vi "Control_Layer.vi"(8 "stop":bool, 10 "Active Axes":bool[](array[boolean]), 11 "Angles":dbl[](array[numeric])=[0.0, 0.0, 0.0, 0.0, 0.0]) -> ()   [LabVIEW 2014]
uses:
  <vilib>/Platform/TimedLoop/XDataNode/timing_clust.ctl
  <vilib>/Platform/TimedLoop/XDataNode/nitl_modes.ctl
  <vilib>/Platform/TimedLoop/XDataNode/wakeup.ctl
  <vilib>/FPGAPlugInAG/cRIO-9068/niLvFpga_Open_cRIO-9068.vi
  <vilib>/rvi/interface/common/dynamic/niFpgaDynamicAddResources.vi
  <vilib>/Utility/error.llb/Error Cluster From Error Code.vi
  <vilib>/rvi/errors/niLvFpgaAdjustHostInterfaceError.vi
  <vilib>/addons/control/pid/pid.llb/PID (DBL).vi
  <vilib>/FPGAPlugInAG/Dynamic/niLvFpga_Close_Dynamic.vi
  <vilib>/rvi/interface/nirviOpenFPGA/nirviOpenFPGA.xnode
  FPGA Bitfiles/MotorControl_FPGATarget_RobotControl_55TRSUIRMao.lvbitx
  <vilib>/rvi/interface/nirviReadWriteControl/nirviReadWriteControl.xnode
  <vilib>/Platform/TimedLoop/XDataNode/XDataNode.xnode
  <vilib>/rvi/interface/nirviCloseFPGA/nirviCloseFPGA.xnode
  <vilib>/rvi/interface/Simulation/niFpgaSimulationCallBeginRW.vi
  NiFpgaLv.dll
  <vilib>/addons/control/pid/NI_PID_pid.lvlib
  <vilib>/Platform/TimedLoop/XDataNode/XDNodeRunTimeDep.lvlib
panel:
  in  "Trapezoidal Move":bool
  out "appended array":dbl[][](array[numeric])
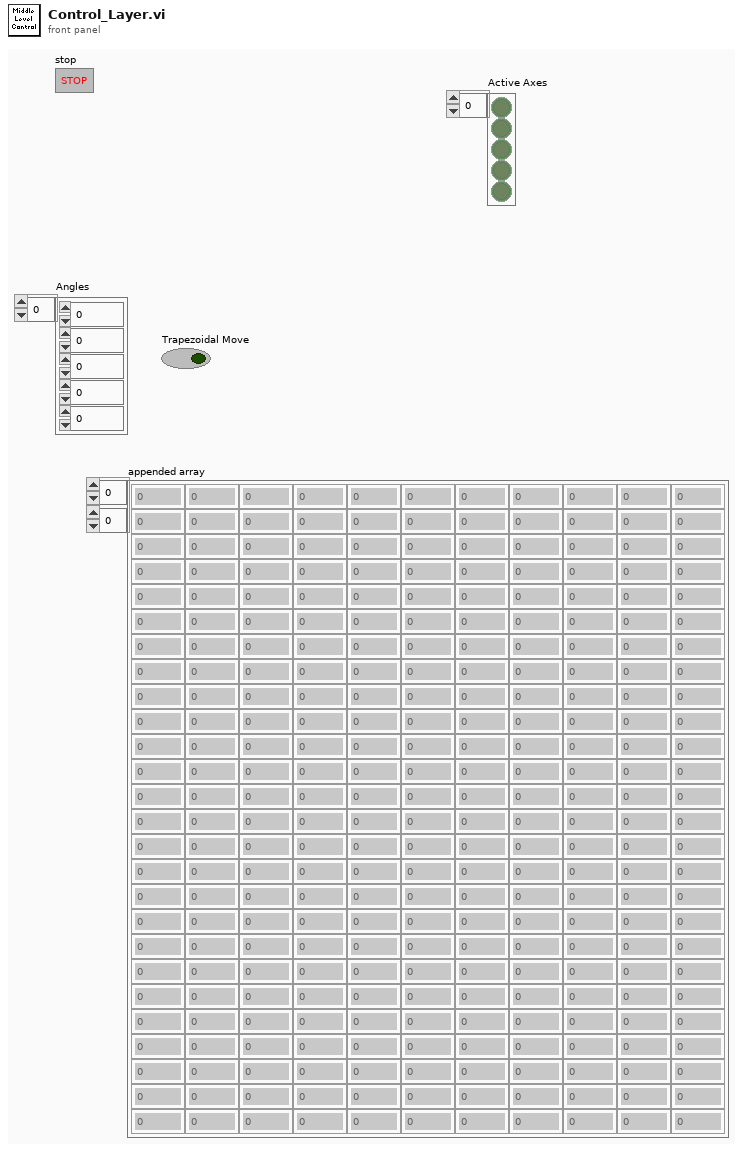
[diagram p1: front panel]
types:
  T1 = typedef "XDNodeRunTimeDep.lvlib/timing_clust.ctl" = cluster{"Expected End [f-1]":u64, "Actual End [f-1]":u64, "Finished Late? [f-1]":bool, "Expected End [i-1]":u64, "Actual End [i-1]":u64, "Finished Late? [i-1]":bool, "Expected Start [i]":u64, "Actual Start [i]":u64, "Expected Start [f]":u64, "Actual Start [f]":u64, "Source Name":string, "Structure Name":string, "Period":i64, "Deadline":i64, "Offset":i64, "Start":i64, "Priority":i32, "Timeout":i32, "Mode":T2, "Wakeup Reason":T3, "Error":errorcluster, "Source Type":string, "Secondary Source Type":string, "Global End Time":u64, "Global Start Time":u64, "Frame Duration":u64, "Iteration Duration":u64, "Assigned CPU":i32, "I/O Scan Engine Mode":u32}
  T2 = typedef "XDNodeRunTimeDep.lvlib/nitl_modes.ctl" = enum32{"No Change", "Process missed periods, maintain original phase", "Discard missed periods, maintain original phase", "Process missed periods, ignore original phase", "Discard missed periods, ignore original phase"}
  T3 = typedef "XDNodeRunTimeDep.lvlib/wakeup.ctl" = enum32{"Normal", "Aborted", "Asynchronous wakeup", "Timing source error", "Timed loop error", "Timeout"}
  T4 = cluster{"Motor 1 Variables":cluster{"Motor 1 P Gains":cluster{"proportional gain (Kc)":dbl, "integral time (Ti, min)":dbl, "derivative time (Td, min)":dbl}, "Motor 1 V Gains":cluster{"proportional gain (Kc)":dbl, "integral time (Ti, min)":dbl, "derivative time (Td, min)":dbl}, "Velocity Limits":cluster{"output high":dbl, "output low":dbl}, "Duty Cycle Limits":cluster{"output high":dbl, "output low":dbl}}, "Motor 2 Variables":cluster{"Motor 2 P Gains":cluster{"proportional gain (Kc)":dbl, "integral time (Ti, min)":dbl, "derivative time (Td, min)":dbl}, "Motor 2 V Gains":cluster{"proportional gain (Kc)":dbl, "integral time (Ti, min)":dbl, "derivative time (Td, min)":dbl}, "Velocity Limits":cluster{"output high":dbl, "output low":dbl}, "Duty Cycle Limits":cluster{"output high":dbl, "output low":dbl}}, "Motor 3 Variables":cluster{"Motor 3 P Gains":cluster{"proportional gain (Kc)":dbl, "integral time (Ti, min)":dbl, "derivative time (Td, min)":dbl}, "Motor 3 V Gains":cluster{"proportional gain (Kc)":dbl, "integral time (Ti, min)":dbl, "derivative time (Td, min)":dbl}, "Velocity Limits":cluster{"output high":dbl, "output low":dbl}, "Duty Cycle Limits":cluster{"output high":dbl, "output low":dbl}}, "Motor 4 Variables":cluster{"Motor 4 P Gains":cluster{"proportional gain (Kc)":dbl, "integral time (Ti, min)":dbl, "derivative time (Td, min)":dbl}, "Motor 4 V Gains":cluster{"proportional gain (Kc)":dbl, "integral time (Ti, min)":dbl, "derivative time (Td, min)":dbl}, "Velocity Limits":cluster{"output high":dbl, "output low":dbl}, "Duty Cycle Limits":cluster{"output high":dbl, "output low":dbl}}, "Motor 5 Variables":cluster{"Motor 5 P Gains":cluster{"proportional gain (Kc)":dbl, "integral time (Ti, min)":dbl, "derivative time (Td, min)":dbl}, "Motor 5 V Gains":cluster{"proportional gain (Kc)":dbl, "integral time (Ti, min)":dbl, "derivative time (Td, min)":dbl}, "Velocity Limits":cluster{"output high":dbl, "output low":dbl}, "Duty Cycle Limits":cluster{"output high":dbl, "output low":dbl}}}
  T5 = cluster{"Motor 1 P Gains":cluster{"proportional gain (Kc)":dbl, "integral time (Ti, min)":dbl, "derivative time (Td, min)":dbl}, "Motor 1 V Gains":cluster{"proportional gain (Kc)":dbl, "integral time (Ti, min)":dbl, "derivative time (Td, min)":dbl}, "Velocity Limits":cluster{"output high":dbl, "output low":dbl}, "Duty Cycle Limits":cluster{"output high":dbl, "output low":dbl}}
  T6 = cluster{"proportional gain (Kc)":dbl, "integral time (Ti, min)":dbl, "derivative time (Td, min)":dbl}
  T7 = cluster{"Motor 2 P Gains":cluster{"proportional gain (Kc)":dbl, "integral time (Ti, min)":dbl, "derivative time (Td, min)":dbl}, "Motor 2 V Gains":cluster{"proportional gain (Kc)":dbl, "integral time (Ti, min)":dbl, "derivative time (Td, min)":dbl}, "Velocity Limits":cluster{"output high":dbl, "output low":dbl}, "Duty Cycle Limits":cluster{"output high":dbl, "output low":dbl}}
  T8 = cluster{"Motor 3 P Gains":cluster{"proportional gain (Kc)":dbl, "integral time (Ti, min)":dbl, "derivative time (Td, min)":dbl}, "Motor 3 V Gains":cluster{"proportional gain (Kc)":dbl, "integral time (Ti, min)":dbl, "derivative time (Td, min)":dbl}, "Velocity Limits":cluster{"output high":dbl, "output low":dbl}, "Duty Cycle Limits":cluster{"output high":dbl, "output low":dbl}}
  T9 = cluster{"Motor 4 P Gains":cluster{"proportional gain (Kc)":dbl, "integral time (Ti, min)":dbl, "derivative time (Td, min)":dbl}, "Motor 4 V Gains":cluster{"proportional gain (Kc)":dbl, "integral time (Ti, min)":dbl, "derivative time (Td, min)":dbl}, "Velocity Limits":cluster{"output high":dbl, "output low":dbl}, "Duty Cycle Limits":cluster{"output high":dbl, "output low":dbl}}
  T10 = cluster{"Motor 5 P Gains":cluster{"proportional gain (Kc)":dbl, "integral time (Ti, min)":dbl, "derivative time (Td, min)":dbl}, "Motor 5 V Gains":cluster{"proportional gain (Kc)":dbl, "integral time (Ti, min)":dbl, "derivative time (Td, min)":dbl}, "Velocity Limits":cluster{"output high":dbl, "output low":dbl}, "Duty Cycle Limits":cluster{"output high":dbl, "output low":dbl}}
  T11 = cluster{"Position (Degrees)":dbl, "Numeric":dbl, "Acceleration":dbl, "Cruise_Velocity":dbl, "Deceleration":dbl, "Time_Accelerate":dbl, "Time_2":dbl, "Time_Total":dbl}
  T12 = cluster{"Acceleration":dbl, "Cruise_Velocity":dbl, "Deceleration":dbl, "Time_Accelerate":dbl, "Time_2":dbl, "Time_Total":dbl}
  T13 = cluster{dbl, "Numeric":dbl, "Acceleration":dbl, "Cruise_Velocity":dbl, "Deceleration":dbl, "Time_Accelerate":dbl, "Time_2":dbl, "Time_Total":dbl}
  T14 = cluster{dbl, dbl, "Acceleration":dbl, "Cruise_Velocity":dbl, "Deceleration":dbl, "Time_Accelerate":dbl, "Time_2":dbl, "Time_Total":dbl}
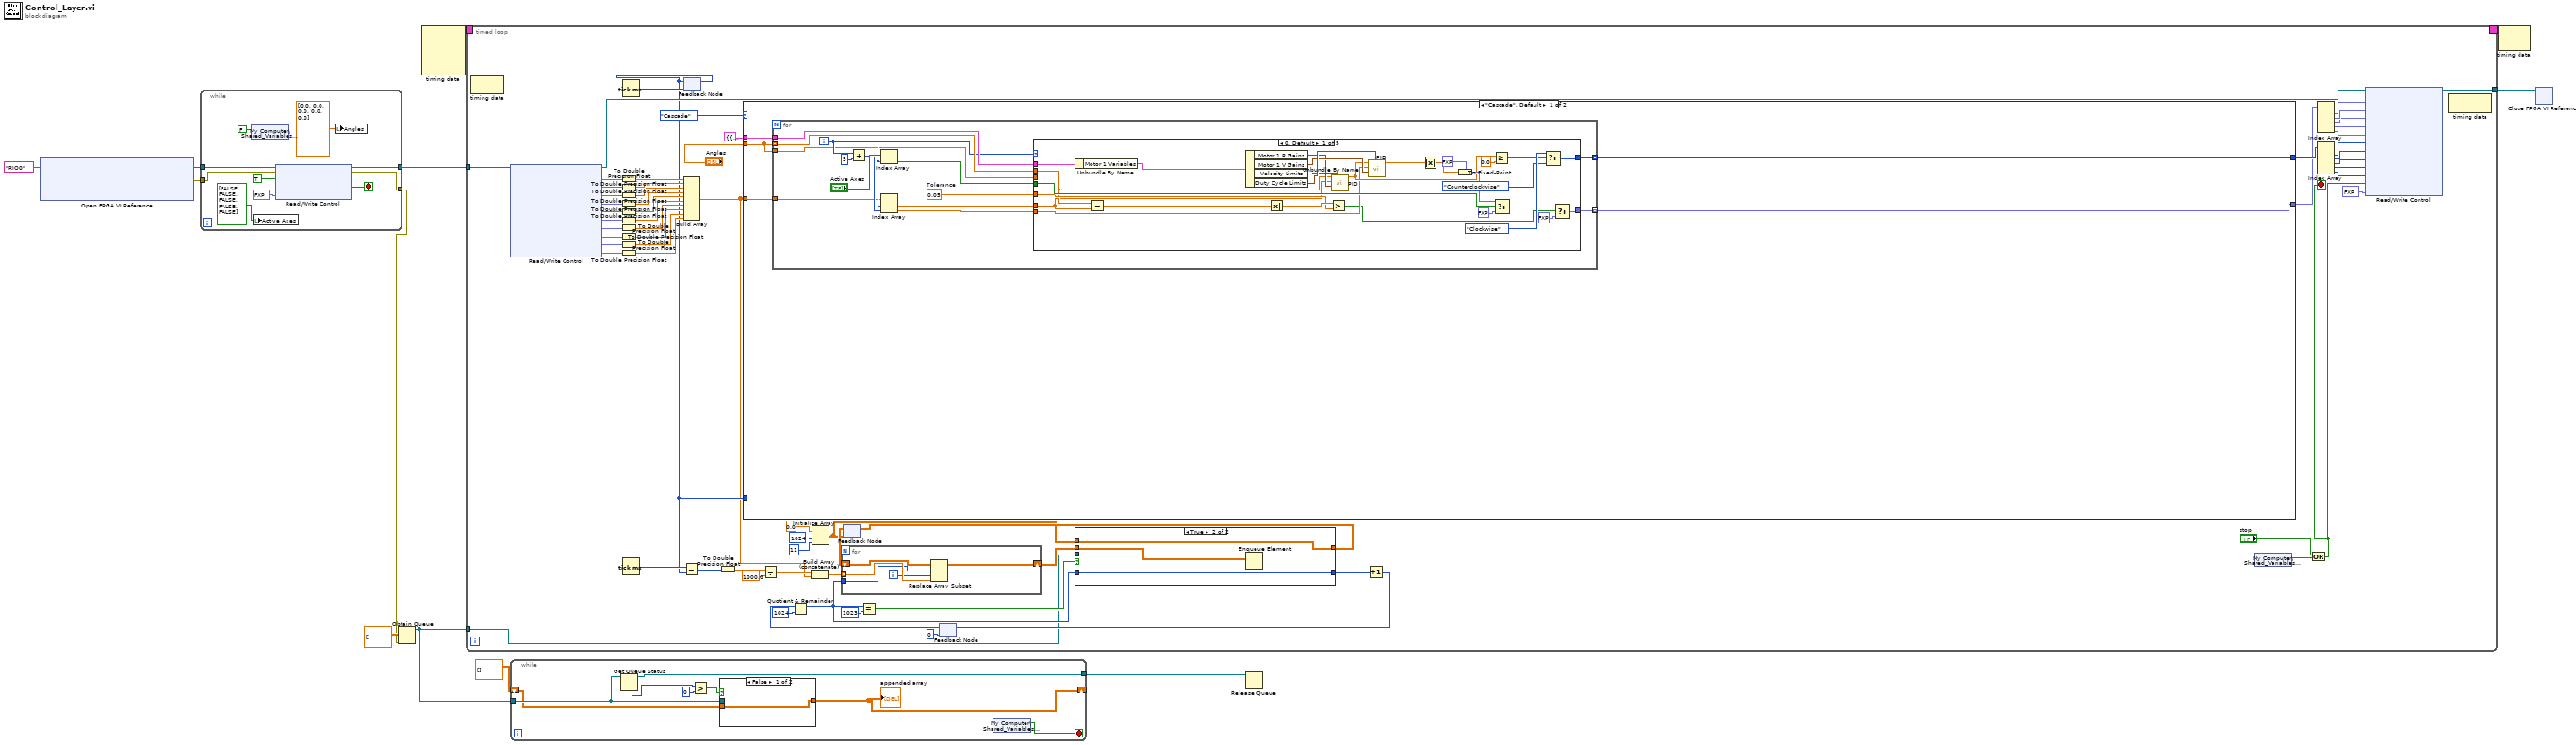
[diagram p0: block diagram]
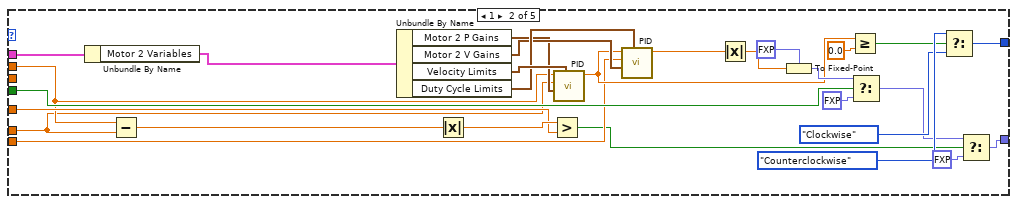
[diagram p2: hidden frame]
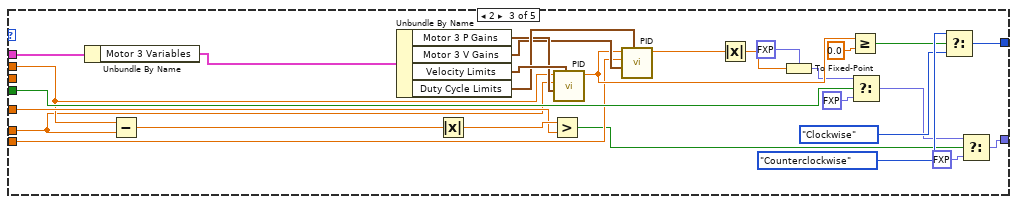
[diagram p3: hidden frame]
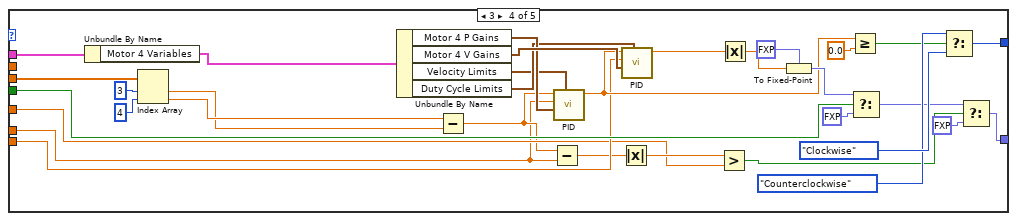
[diagram p4: hidden frame]
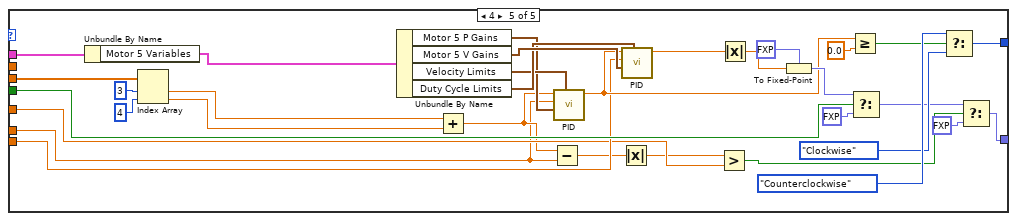
[diagram p5: hidden frame]
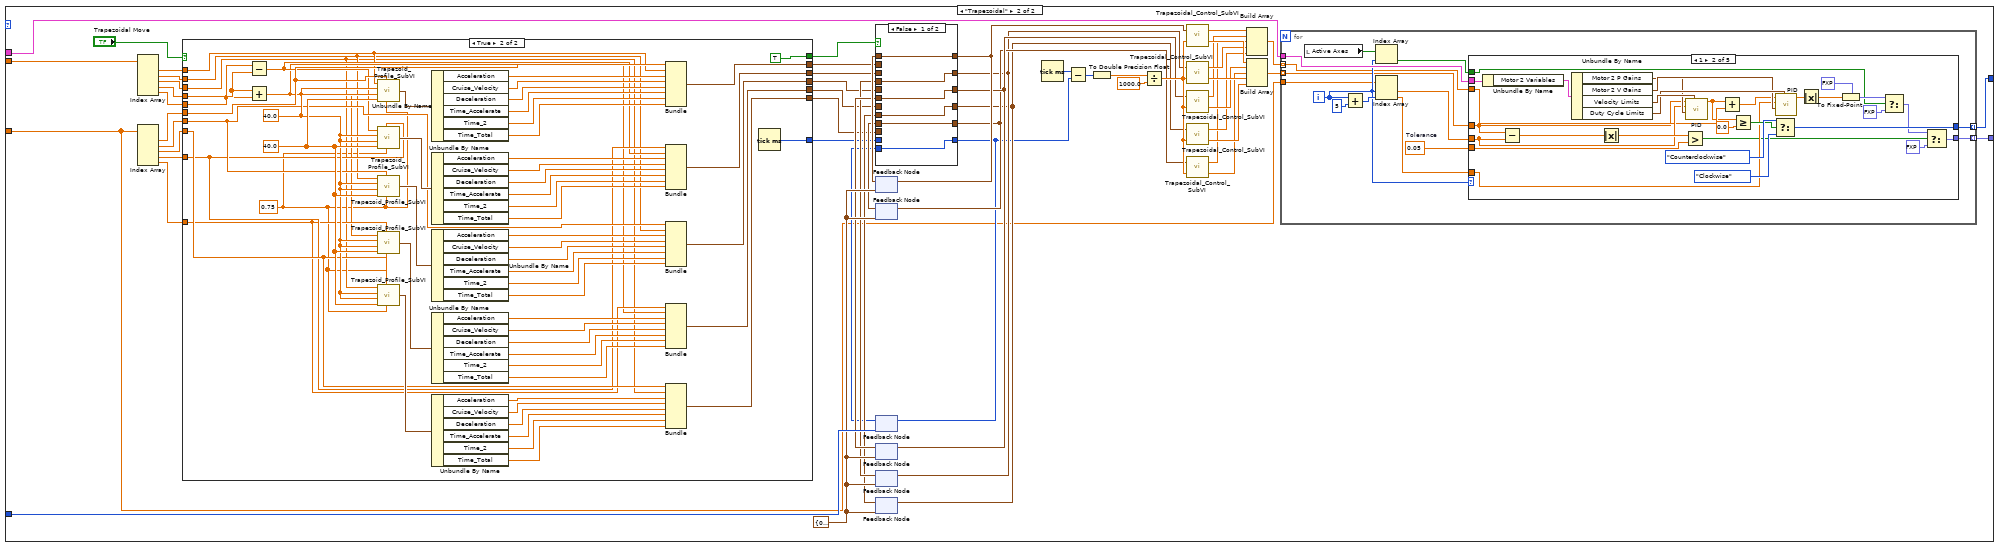
[diagram p6: hidden frame]
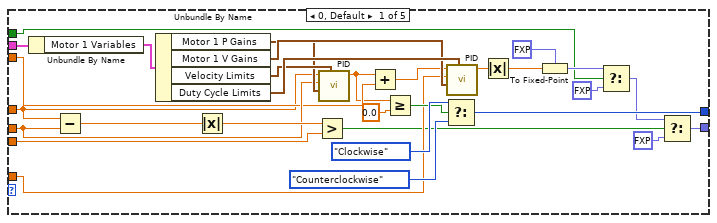
[diagram p7: hidden frame]
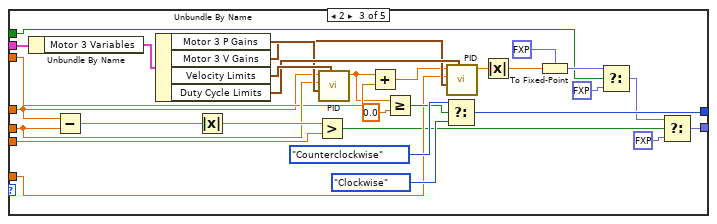
[diagram p8: hidden frame]
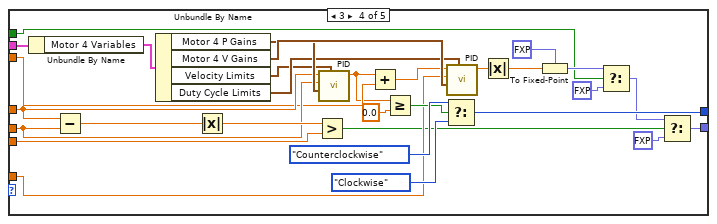
[diagram p9: hidden frame]
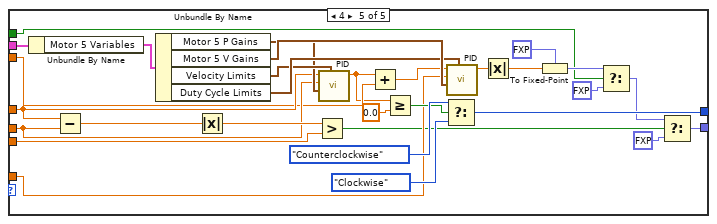
[diagram p10: hidden frame]
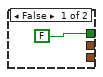
[diagram p11: hidden frame]
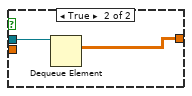
[diagram p14: hidden frame]
diagram:
  n1 = xnode "Open FPGA VI Reference"("resource name"=tag "RIO0") -> ("FPGA VI Reference Out"=w11:refnum<k20>, "error out"=w2:errorcluster)  [unwired: 1 in]
  n2 = while {
    tunnel: w11 -> [w22]
    tunnel: [w19] -> w6
    tunnel: w2 -> [w14]
    tunnel: [w13] -> w1
    stop <- w20 stop-if-true
    n3 = shared-variable "My Computer\\Shared_Variables.lvlib\\Stop"(FALSE ("Stop")) -> ()  [unwired: 1 in, 1 out]
    n4 = local write "Active Axes"(bool[] [FALSE, FALSE, FALSE, FALSE, FALSE] ("Active Axes")) -> ()
    n5 = xnode "Read/Write Control"("FPGA VI Reference In"=w22, "error in"=w14, "Go"=TRUE, "Velocity Interval (uSec)"=fxp<+/-,40,24> 5000.0) -> ("FPGA VI Reference Out"=w19:refnum<k20>, "error out"=w13:errorcluster, "Homed"=w20:bool)
    n6 = local write "Angles"(dbl[] [0.0, 0.0, 0.0, 0.0, 0.0] ("Angles")) -> ()
  }
  n7 = Obtain Queue(element data type=dbl[][] [], error in (no error)=w1) -> (queue out=w9:refnum<queue>)  [unwired: 3 in, 2 out]
  n8 = node-c288() -> (w4:T1)  [unwired: 4 in]
  n9 = timed-loop {
    tunnel: [w89] -> w12
    tunnel: w6 -> [w87]
    tunnel: w9 -> [w46]
    timing: w4 -> [_]
    timing-out: [_] -> w3
    stop <- w25 stop-if-true
    n10 = node-c288() -> ()  [unwired: 1 in, 1 out]
    n11 = xnode "Read/Write Control"("FPGA VI Reference In"=w87) -> ("FPGA VI Reference Out"=w82:refnum<k20>, "Position (Degrees)"=w81:fxp<+/-,40,24>, "Position (Degrees) 2"=w80:fxp<+/-,40,24>, "Position (Degrees) 3"=w79:fxp<+/-,40,24>, "Position (Degrees) 4"=w78:fxp<+/-,40,24>, "Position (Degrees) 5"=w77:fxp<+/-,40,24>, "Velocity (Degrees/Second)"=w76:fxp<+/-,40,24>, "Velocity (Degrees/Second) 2"=w75:fxp<+/-,40,24>, "Velocity (Degrees/Second) 3"=w74:fxp<+/-,40,24>, "Velocity (Degrees/Second) 4"=w73:fxp<+/-,40,24>, "Velocity (Degrees/Second) 5"=w72:fxp<+/-,40,24>)  [unwired: 1 in, 1 out]
    n12 = To Double Precision Float(number=w81) -> (double precision float=w64:dbl)
    n13 = To Double Precision Float(number=w80) -> (double precision float=w63:dbl)
    n14 = To Double Precision Float(number=w79) -> (double precision float=w62:dbl)
    n15 = To Double Precision Float(number=w78) -> (double precision float=w61:dbl)
    n16 = To Double Precision Float(number=w77) -> (double precision float=w60:dbl)
    n17 = To Double Precision Float(number=w76) -> (double precision float=w59:dbl)
    n18 = To Double Precision Float(number=w75) -> (double precision float=w58:dbl)
    n19 = To Double Precision Float(number=w74) -> (double precision float=w57:dbl)
    n20 = To Double Precision Float(number=w73) -> (double precision float=w56:dbl)
    n21 = To Double Precision Float(number=w72) -> (double precision float=w55:dbl)
    n22 = Tick Count (ms)() -> (millisecond timer value=w44:u32)
    n23 = Tick Count (ms)() -> (millisecond timer value=w86:u32)
    n24 = Build Array(w64, w63, w62, w61, w60, w59, w58, w57, w56, w55) -> (w39:dbl[])
    n25 = feedback #1(w44) -> (w43:u32)
    n26 = Subtract(x=w86, y=w43) -> (x-y=w85:u32)
    n27 = feedback-in #1(w43) -> ()
    n28 = To Double Precision Float(number=w85) -> (double precision float=w83:dbl)
    n29 = case shown="\"Cascade\", Default" enum16{"Cascade", "Trapezoidal"}."Cascade" {
      tunnel: w43 -> [_ w314]
      tunnel: T4 {"Motor 1 Variables"={"Motor 1 P Gains"={"proportional gain (Kc)"=3.0, "integral time (Ti, min)"=0.0, "derivative time (Td, min)"=0.0}, "Motor 1 V Gains"={"proportional gain (Kc)"=0.001, "integral time (Ti, min)"=0.0001, "derivative time (Td, min)"=0.0}, "Velocity Limits"={"output high"=40.0, "output low"=-40.0}, "Duty Cycle Limits"={"output high"=0.6, "output low"=-0.6}}, "Motor 2 Variables"={"Motor 2 P Gains"={"proportional gain (Kc)"=2.0, "integral time (Ti, min)"=0.0, "derivative time (Td, min)"=0.0}, "Motor 2 V Gains"={"proportional gain (Kc)"=0.002, "integral time (Ti, min)"=0.0003, "derivative time (Td, min)"=0.0}, "Velocity Limits"={"output high"=40.0, "output low"=-40.0}, "Duty Cycle Limits"={"output high"=0.6, "output low"=-0.6}}, "Motor 3 Variables"={"Motor 3 P Gains"={"proportional gain (Kc)"=2.0, "integral time (Ti, min)"=0.0, "derivative time (Td, min)"=0.0}, "Motor 3 V Gains"={"proportional gain (Kc)"=0.004, "integral time (Ti, min)"=0.0003, "derivative time (Td, min)"=0.0}, "Velocity Limits"={"output high"=40.0, "output low"=-40.0}, "Duty Cycle Limits"={"output high"=0.6, "output low"=-0.6}}, "Motor 4 Variables"={"Motor 4 P Gains"={"proportional gain (Kc)"=3.0, "integral time (Ti, min)"=0.0, "derivative time (Td, min)"=0.0}, "Motor 4 V Gains"={"proportional gain (Kc)"=0.0004, "integral time (Ti, min)"=0.0001, "derivative time (Td, min)"=0.0}, "Velocity Limits"={"output high"=40.0, "output low"=-40.0}, "Duty Cycle Limits"={"output high"=0.6, "output low"=-0.6}}, "Motor 5 Variables"={"Motor 5 P Gains"={"proportional gain (Kc)"=3.0, "integral time (Ti, min)"=0.0, "derivative time (Td, min)"=0.0}, "Motor 5 V Gains"={"proportional gain (Kc)"=0.0004, "integral time (Ti, min)"=0.0001, "derivative time (Td, min)"=0.0}, "Velocity Limits"={"output high"=40.0, "output low"=-40.0}, "Duty Cycle Limits"={"output high"=0.6, "output low"=-0.6}}} ("Motor Variables") -> [w95 w275]
      tunnel: "Angles" -> [w94 w282]
      tunnel: w39 -> [w96 w276]
      tunnel: [w93 w269] -> w38
      tunnel: [w92 w270] -> w32
      frame "Cascade", Default {
        n30 = for {
          tunnel: w94 -> [w109] mode=indexing
          tunnel: w96 -> [w100]
          tunnel: w95 -> [w110]
          tunnel: [w108] -> w93 mode=indexing
          tunnel: [w107] -> w92 mode=indexing
          tunnel: w94 -> [w98]
          i -> [w102]
          w97 = 0.05  # Tolerance
          n31 = Add(x=w102, y=5) -> (x+y=w103:i32)
          n32 = Index Array(array="Active Axes", index=w102) -> (element=w105:bool)
          n33 = Index Array(array=w100, index #1=w102, index #2=w103) -> (element #1=w101:dbl, element #2=w99:dbl)
          n34 = case shown="0, Default" w102 {
            tunnel: w110 -> [w124 w153 w180 w213 w246]
            tunnel: w109 -> [w112 w140 w168 _ _]
            tunnel: [w123 w152 w179 w212 w245] -> w108
            tunnel: [w116 w141 w169 w197 w230] -> w107
            tunnel: w105 -> [w122 w151 w178 w211 w244]
            tunnel: w101 -> [w111 w139 w167 w195 w228]
            tunnel: w99 -> [w120 w148 w176 w209 w242]
            tunnel: w98 -> [_ _ _ w208 w239]
            tunnel: w97 -> [w114 w143 w171 w199 w234]
            frame 0, Default {
              n35 = Unbundle By Name(w124) -> ("Motor 1 Variables"=w125:T5)
              n36 = Subtract(x=w112, y=w111) -> (x-y=w113:dbl)
              n37 = Unbundle By Name(w125) -> ("Motor 1 P Gains"=w130:T6, "Motor 1 V Gains"=w131:T6, "Velocity Limits"=w132:cluster{"output high":dbl, "output low":dbl}, "Duty Cycle Limits"=w133:cluster{"output high":dbl, "output low":dbl})
              n38 = Absolute Value(x=w113) -> (abs(x)=w115:dbl)
              n39 = Greater?(x=w115, y=w114) -> (0:w118:bool)
              n40 = call-poly <vilib>:"PID.vi"("output range"=w132, "PID gains"=w130, "process variable"=w111, "setpoint"=w112) -> ("output"=w127:dbl)  [unwired: 6 in, 1 out]
              n41 = call-poly <vilib>:"PID.vi"("output range"=w133, "PID gains"=w131, "process variable"=w120, "setpoint"=w127) -> ("output"=w128:dbl)  [unwired: 6 in, 1 out]
              n42 = Absolute Value(x=w128) -> (abs(x)=w129:dbl)
              n43 = To Fixed-Point(fixed-point type=fxp<+,32,0> 0.0 ("Duty Cycle 1"), number=w129) -> (fixed-point=w135:fxp<+,32,0>)
              n44 = Greater Or Equal?(x=w127, y=0.0) -> (x >= y?=w136:bool)
              n45 = Select(t=w135, s=w122, f=fxp<+,32,0> 0.0 ("Duty Cycle 1")) -> (s? t:f=w117:fxp<+,32,0>)
              n46 = Select(t=enum8{"Clockwise", "Counterclockwise"}."Clockwise" ("Mod1/Drive Direction"), s=w136, f=enum8{"Clockwise", "Counterclockwise"}."Counterclockwise" ("Mod1/Drive Direction")) -> (s? t:f=w123:enum8{"Clockwise", "Counterclockwise"})
              n47 = Select(t=w117, s=w118, f=fxp<+,32,0> 0.0 ("Duty Cycle 1")) -> (s? t:f=w116:fxp<+,32,0>)
            }
            frame 1 {
              n48 = Unbundle By Name(w153) -> ("Motor 2 Variables"=w154:T7)
              n49 = Subtract(x=w140, y=w139) -> (x-y=w145:dbl)
              n50 = Unbundle By Name(w154) -> ("Motor 2 P Gains"=w158:T6, "Motor 2 V Gains"=w159:T6, "Velocity Limits"=w161:cluster{"output high":dbl, "output low":dbl}, "Duty Cycle Limits"=w160:cluster{"output high":dbl, "output low":dbl})
              n51 = Absolute Value(x=w145) -> (abs(x)=w144:dbl)
              n52 = Greater?(x=w144, y=w143) -> (0:w146:bool)
              n53 = call-poly <vilib>:"PID.vi"("output range"=w161, "PID gains"=w158, "process variable"=w139, "setpoint"=w140) -> ("output"=w149:dbl)  [unwired: 6 in, 1 out]
              n54 = call-poly <vilib>:"PID.vi"("output range"=w160, "PID gains"=w159, "process variable"=w148, "setpoint"=w149) -> ("output"=w156:dbl)  [unwired: 6 in, 1 out]
              n55 = Absolute Value(x=w156) -> (abs(x)=w157:dbl)
              n56 = To Fixed-Point(fixed-point type=fxp<+,32,0> 0.0 ("Duty Cycle 1"), number=w157) -> (fixed-point=w163:fxp<+,32,0>)
              n57 = Greater Or Equal?(x=w149, y=0.0) -> (x >= y?=w164:bool)
              n58 = Select(t=w163, s=w151, f=fxp<+,32,0> 0.0 ("Duty Cycle 1")) -> (s? t:f=w142:fxp<+,32,0>)
              n59 = Select(t=enum8{"Clockwise", "Counterclockwise"}."Counterclockwise" ("Mod1/Drive Direction"), s=w164, f=enum8{"Clockwise", "Counterclockwise"}."Clockwise" ("Mod1/Drive Direction")) -> (s? t:f=w152:enum8{"Clockwise", "Counterclockwise"})
              n60 = Select(t=w142, s=w146, f=fxp<+,32,0> 0.0 ("Duty Cycle 1")) -> (s? t:f=w141:fxp<+,32,0>)
            }
            frame 2 {
              n61 = Unbundle By Name(w180) -> ("Motor 3 Variables"=w181:T8)
              n62 = Subtract(x=w168, y=w167) -> (x-y=w173:dbl)
              n63 = Unbundle By Name(w181) -> ("Motor 3 P Gains"=w189:T6, "Motor 3 V Gains"=w188:T6, "Velocity Limits"=w191:cluster{"output high":dbl, "output low":dbl}, "Duty Cycle Limits"=w190:cluster{"output high":dbl, "output low":dbl})
              n64 = Absolute Value(x=w173) -> (abs(x)=w172:dbl)
              n65 = Greater?(x=w172, y=w171) -> (0:w174:bool)
              n66 = call-poly <vilib>:"PID.vi"("output range"=w191, "PID gains"=w189, "process variable"=w167, "setpoint"=w168) -> ("output"=w185:dbl)  [unwired: 6 in, 1 out]
              n67 = call-poly <vilib>:"PID.vi"("output range"=w190, "PID gains"=w188, "process variable"=w176, "setpoint"=w185) -> ("output"=w186:dbl)  [unwired: 6 in, 1 out]
              n68 = Absolute Value(x=w186) -> (abs(x)=w187:dbl)
              n69 = To Fixed-Point(fixed-point type=fxp<+,32,0> 0.0 ("Duty Cycle 1"), number=w187) -> (fixed-point=w182:fxp<+,32,0>)
              n70 = Greater Or Equal?(x=w185, y=0.0) -> (x >= y?=w192:bool)
              n71 = Select(t=w182, s=w178, f=fxp<+,32,0> 0.0 ("Duty Cycle 1")) -> (s? t:f=w170:fxp<+,32,0>)
              n72 = Select(t=enum8{"Clockwise", "Counterclockwise"}."Counterclockwise" ("Mod1/Drive Direction"), s=w192, f=enum8{"Clockwise", "Counterclockwise"}."Clockwise" ("Mod1/Drive Direction")) -> (s? t:f=w179:enum8{"Clockwise", "Counterclockwise"})
              n73 = Select(t=w170, s=w174, f=fxp<+,32,0> 0.0 ("Duty Cycle 1")) -> (s? t:f=w169:fxp<+,32,0>)
            }
            frame 3 {
              n74 = Unbundle By Name(w213) -> ("Motor 4 Variables"=w214:T9)
              n75 = Index Array(array=w208, index #1=3 ("index"), index #2=4 ("index")) -> (element #1=w204:dbl, element #2=w205:dbl)
              n76 = Unbundle By Name(w214) -> ("Motor 4 P Gains"=w221:T6, "Motor 4 V Gains"=w222:T6, "Velocity Limits"=w219:cluster{"output high":dbl, "output low":dbl}, "Duty Cycle Limits"=w220:cluster{"output high":dbl, "output low":dbl})
              n77 = Subtract(x=w205, y=w204) -> (x-y=w196:dbl)
              n78 = Subtract(x=w196, y=w195) -> (x-y=w201:dbl)
              n79 = call-poly <vilib>:"PID.vi"("output range"=w219, "PID gains"=w221, "process variable"=w195, "setpoint"=w196) -> ("output"=w216:dbl)  [unwired: 6 in, 1 out]
              n80 = Absolute Value(x=w201) -> (abs(x)=w200:dbl)
              n81 = call-poly <vilib>:"PID.vi"("output range"=w220, "PID gains"=w222, "process variable"=w209, "setpoint"=w216) -> ("output"=w217:dbl)  [unwired: 6 in, 1 out]
              n82 = Greater?(x=w200, y=w199) -> (0:w202:bool)
              n83 = Absolute Value(x=w217) -> (abs(x)=w218:dbl)
              n84 = To Fixed-Point(fixed-point type=fxp<+,32,0> 0.0 ("Duty Cycle 1"), number=w218) -> (fixed-point=w224:fxp<+,32,0>)
              n85 = Greater Or Equal?(x=w216, y=0.0) -> (x >= y?=w225:bool)
              n86 = Select(t=w224, s=w211, f=fxp<+,32,0> 0.0 ("Duty Cycle 1")) -> (s? t:f=w198:fxp<+,32,0>)
              n87 = Select(t=enum8{"Clockwise", "Counterclockwise"}."Counterclockwise" ("Mod1/Drive Direction"), s=w225, f=enum8{"Clockwise", "Counterclockwise"}."Clockwise" ("Mod1/Drive Direction")) -> (s? t:f=w212:enum8{"Clockwise", "Counterclockwise"})
              n88 = Select(t=w198, s=w202, f=fxp<+,32,0> 0.0 ("Duty Cycle 1")) -> (s? t:f=w197:fxp<+,32,0>)
            }
            frame 4 {
              n89 = Unbundle By Name(w246) -> ("Motor 5 Variables"=w247:T10)
              n90 = Index Array(array=w239, index #1=3 ("index"), index #2=4 ("index")) -> (element #1=w238:dbl, element #2=w237:dbl)
              n91 = Unbundle By Name(w247) -> ("Motor 5 P Gains"=w252:T6, "Motor 5 V Gains"=w255:T6, "Velocity Limits"=w253:cluster{"output high":dbl, "output low":dbl}, "Duty Cycle Limits"=w254:cluster{"output high":dbl, "output low":dbl})
              n92 = Add(x=w238, y=w237) -> (x+y=w229:dbl)
              n93 = Subtract(x=w229, y=w228) -> (x-y=w232:dbl)
              n94 = call-poly <vilib>:"PID.vi"("output range"=w253, "PID gains"=w252, "process variable"=w228, "setpoint"=w229) -> ("output"=w249:dbl)  [unwired: 6 in, 1 out]
              n95 = Absolute Value(x=w232) -> (abs(x)=w233:dbl)
              n96 = call-poly <vilib>:"PID.vi"("output range"=w254, "PID gains"=w255, "process variable"=w242, "setpoint"=w249) -> ("output"=w250:dbl)  [unwired: 6 in, 1 out]
              n97 = Greater?(x=w233, y=w234) -> (0:w235:bool)
              n98 = Absolute Value(x=w250) -> (abs(x)=w251:dbl)
              n99 = To Fixed-Point(fixed-point type=fxp<+,32,0> 0.0 ("Duty Cycle 1"), number=w251) -> (fixed-point=w257:fxp<+,32,0>)
              n100 = Greater Or Equal?(x=w249, y=0.0) -> (x >= y?=w258:bool)
              n101 = Select(t=w257, s=w244, f=fxp<+,32,0> 0.0 ("Duty Cycle 1")) -> (s? t:f=w231:fxp<+,32,0>)
              n102 = Select(t=enum8{"Clockwise", "Counterclockwise"}."Counterclockwise" ("Mod1/Drive Direction"), s=w258, f=enum8{"Clockwise", "Counterclockwise"}."Clockwise" ("Mod1/Drive Direction")) -> (s? t:f=w245:enum8{"Clockwise", "Counterclockwise"})
              n103 = Select(t=w231, s=w235, f=fxp<+,32,0> 0.0 ("Duty Cycle 1")) -> (s? t:f=w230:fxp<+,32,0>)
            }
          }
        }
      }
      frame "Trapezoidal" {
        w313 = T11 {"Position (Degrees)"=0.0, "Numeric"=0.0, "Acceleration"=0.0, "Cruise_Velocity"=0.0, "Deceleration"=0.0, "Time_Accelerate"=0.0, "Time_2"=0.0, "Time_Total"=0.0}
        n104 = Index Array(array=w282) -> (element #1=w281:dbl, element #2=w280:dbl, element #3=w279:dbl, element #4=w278:dbl, element #5=w277:dbl)  [unwired: 5 in]
        n105 = Index Array(array=w276) -> (element #1=w287:dbl, element #2=w286:dbl, element #3=w285:dbl, element #4=w284:dbl, element #5=w283:dbl)  [unwired: 5 in]
        n106 = case shown="True" "Trapezoidal Move" {
          tunnel: [_ w527] -> w310
          tunnel: [_ w498] -> w305
          tunnel: [_ w497] -> w304
          tunnel: [_ w496] -> w303
          tunnel: [_ w495] -> w302
          tunnel: [FALSE TRUE] -> w312
          tunnel: [_ w493] -> w301
          tunnel: w287 -> [_ w492]
          tunnel: w286 -> [_ w491]
          tunnel: w285 -> [_ w490]
          tunnel: w284 -> [_ w489]
          tunnel: w283 -> [_ w488]
          tunnel: w281 -> [_ w485]
          tunnel: w280 -> [_ w484]
          tunnel: w279 -> [_ w483]
          tunnel: w278 -> [_ w482]
          tunnel: w277 -> [_ w481]
          frame False {
          }
          frame True {
            w535 = 40.0 ("Acceleration")
            w536 = 40.0 ("Vcruise")
            w480 = 0.75 ("MinFrac_Cruise")
            n107 = Subtract(x=w481, y=w482) -> (x-y=w487:dbl)
            n108 = Add(x=w482, y=w481) -> (x+y=w486:dbl)
            n109 = call "Trapezoid_Profile_SubVI.vi"("MinFrac_Cruise"=w480, "Init_Position"=w492, "Vcruise"=w536, "Deceleration"=w535, "Acceleration"=w535, "Final Position"=w485) -> ("Outputs"=w534:T12)
            n110 = call "Trapezoid_Profile_SubVI.vi"("MinFrac_Cruise"=w480, "Init_Position"=w489, "Vcruise"=w536, "Deceleration"=w535, "Acceleration"=w535, "Final Position"=w487) -> ("Outputs"=w501:T12)
            n111 = call "Trapezoid_Profile_SubVI.vi"("MinFrac_Cruise"=w480, "Init_Position"=w491, "Vcruise"=w536, "Deceleration"=w535, "Acceleration"=w535, "Final Position"=w484) -> ("Outputs"=w499:T12)
            n112 = call "Trapezoid_Profile_SubVI.vi"("MinFrac_Cruise"=w480, "Init_Position"=w488, "Vcruise"=w536, "Deceleration"=w535, "Acceleration"=w535, "Final Position"=w486) -> ("Outputs"=w502:T12)
            n113 = call "Trapezoid_Profile_SubVI.vi"("MinFrac_Cruise"=w480, "Init_Position"=w490, "Vcruise"=w536, "Deceleration"=w535, "Acceleration"=w535, "Final Position"=w483) -> ("Outputs"=w500:T12)
            n114 = Unbundle By Name(w534) -> ("Acceleration"=w528:dbl, "Cruise_Velocity"=w529:dbl, "Deceleration"=w530:dbl, "Time_Accelerate"=w531:dbl, "Time_2"=w532:dbl, "Time_Total"=w533:dbl)
            n115 = Unbundle By Name(w501) -> ("Acceleration"=w514:dbl, "Cruise_Velocity"=w513:dbl, "Deceleration"=w512:dbl, "Time_Accelerate"=w511:dbl, "Time_2"=w510:dbl, "Time_Total"=w509:dbl)
            n116 = Unbundle By Name(w499) -> ("Acceleration"=w526:dbl, "Cruise_Velocity"=w525:dbl, "Deceleration"=w524:dbl, "Time_Accelerate"=w523:dbl, "Time_2"=w522:dbl, "Time_Total"=w521:dbl)
            n117 = Unbundle By Name(w502) -> ("Acceleration"=w503:dbl, "Cruise_Velocity"=w504:dbl, "Deceleration"=w505:dbl, "Time_Accelerate"=w506:dbl, "Time_2"=w507:dbl, "Time_Total"=w508:dbl)
            n118 = Unbundle By Name(w500) -> ("Acceleration"=w515:dbl, "Cruise_Velocity"=w516:dbl, "Deceleration"=w517:dbl, "Time_Accelerate"=w518:dbl, "Time_2"=w519:dbl, "Time_Total"=w520:dbl)
            n119 = Bundle(w492, "Numeric"=w485, "Acceleration"=w528, "Cruise_Velocity"=w529, "Deceleration"=w530, "Time_Accelerate"=w531, "Time_2"=w532, "Time_Total"=w533) -> (w527:T13)  [unwired: 1 in]
            n120 = Bundle(w489, w487, "Acceleration"=w514, "Cruise_Velocity"=w513, "Deceleration"=w512, "Time_Accelerate"=w511, "Time_2"=w510, "Time_Total"=w509) -> (w496:T14)  [unwired: 1 in]
            n121 = Bundle(w491, "Numeric"=w484, "Acceleration"=w526, "Cruise_Velocity"=w525, "Deceleration"=w524, "Time_Accelerate"=w523, "Time_2"=w522, "Time_Total"=w521) -> (w498:T13)  [unwired: 1 in]
            n122 = Bundle(w488, w486, "Acceleration"=w503, "Cruise_Velocity"=w504, "Deceleration"=w505, "Time_Accelerate"=w506, "Time_2"=w507, "Time_Total"=w508) -> (w495:T14)  [unwired: 1 in]
            n123 = Bundle(w490, "Numeric"=w483, "Acceleration"=w515, "Cruise_Velocity"=w516, "Deceleration"=w517, "Time_Accelerate"=w518, "Time_2"=w519, "Time_Total"=w520) -> (w497:T13)  [unwired: 1 in]
            n124 = Tick Count (ms)() -> (millisecond timer value=w493:u32)
          }
        }
        n125 = feedback #2(w313) -> (w311:T11)
        n126 = feedback #3(w313) -> (w308:T11)
        n127 = feedback #4(w314) -> (w300:u32)
        n128 = feedback #5(w313) -> (w309:T11)
        n129 = feedback #6(w313) -> (w307:T11)
        n130 = feedback #7(w313) -> (w306:T11)
        n131 = case shown="False" w312 {
          tunnel: w311 -> [w542 _]
          tunnel: [w542 w548] -> w295
          tunnel: w310 -> [_ w548]
          tunnel: [w541 w547] -> w294
          tunnel: [w540 w546] -> w293
          tunnel: [w539 w545] -> w292
          tunnel: [w538 w544] -> w291
          tunnel: w309 -> [w541 _]
          tunnel: w308 -> [w540 _]
          tunnel: w307 -> [w539 _]
          tunnel: w306 -> [w538 _]
          tunnel: w305 -> [_ w547]
          tunnel: w304 -> [_ w546]
          tunnel: w303 -> [_ w545]
          tunnel: w302 -> [_ w544]
          tunnel: w301 -> [_ w543]
          tunnel: w300 -> [w537 _]
          tunnel: [w537 w543] -> w289
          frame False {
          }
          frame True {
          }
        }
        n132 = feedback-in #2(w295) -> ()
        n133 = feedback-in #3(w293) -> ()
        n134 = feedback-in #4(w289) -> ()
        n135 = feedback-in #5(w294) -> ()
        n136 = feedback-in #6(w292) -> ()
        n137 = feedback-in #7(w291) -> ()
        n138 = Tick Count (ms)() -> (millisecond timer value=w290:u32)
        n139 = Subtract(x=w290, y=w289) -> (x-y=w298:u32)
        n140 = To Double Precision Float(number=w298) -> (double precision float=w297:dbl)
        n141 = Divide(x=w297, y=1000.0) -> (x/y=w296:dbl)
        n142 = call "Trapezoidal_Control_SubVI.vi"("Current_Time"=w296, "Inputs"=w295) -> ("pSetProfile"=w274:dbl, "vSetProfile"=w273:dbl)
        n143 = call "Trapezoidal_Control_SubVI.vi"("Current_Time"=w296, "Inputs"=w292) -> ("pSetProfile"=w267:dbl, "vSetProfile"=w268:dbl)
        n144 = call "Trapezoidal_Control_SubVI.vi"("Current_Time"=w296, "Inputs"=w294) -> ("pSetProfile"=w265:dbl, "vSetProfile"=w266:dbl)
        n145 = call "Trapezoidal_Control_SubVI.vi"("Current_Time"=w296, "Inputs"=w291) -> ("pSetProfile"=w263:dbl, "vSetProfile"=w264:dbl)
        n146 = call "Trapezoidal_Control_SubVI.vi"("Current_Time"=w296, "Inputs"=w293) -> ("pSetProfile"=w261:dbl, "vSetProfile"=w262:dbl)
        n147 = Build Array(w273, w266, w262, w268, w264) -> (w271:dbl[])
        n148 = Build Array(w274, w265, w261, w267, w263) -> (w272:dbl[])
        n149 = for {
          tunnel: w276 -> [w320]
          tunnel: w275 -> [w328]
          tunnel: [w327] -> w269 mode=indexing
          tunnel: [w326] -> w270 mode=indexing
          tunnel: w272 -> [w316] mode=indexing
          tunnel: w271 -> [w315] mode=indexing
          i -> [w322]
          w318 = 0.05  # Tolerance
          n150 = local read "Active Axes"() -> (w317:bool[])
          n151 = Add(x=w322, y=5) -> (x+y=w323:i32)
          n152 = Index Array(array=w317, index=w322) -> (element=w325:bool)
          n153 = Index Array(array=w320, index #1=w322, index #2=w323) -> (element #1=w321:dbl, element #2=w319:dbl)
          n154 = case shown="1" w322 {
            tunnel: w328 -> [w345 w375 w405 w435 w465]
            tunnel: [w344 w374 w404 w434 w464] -> w327
            tunnel: [w337 w364 w394 w424 w454] -> w326
            tunnel: w325 -> [w343 w373 w403 w433 w463]
            tunnel: w321 -> [w333 w363 w393 w423 w453]
            tunnel: w319 -> [w341 w371 w401 w431 w461]
            tunnel: w318 -> [w335 w366 w396 w426 w458]
            tunnel: w316 -> [w329 w359 w389 w422 w452]
            tunnel: w315 -> [w332 w362 w392 w421 w451]
            frame 0, Default {
              n155 = Unbundle By Name(w345) -> ("Motor 1 Variables"=w346:T5)
              n156 = Subtract(x=w329, y=w333) -> (x-y=w334:dbl)
              n157 = Unbundle By Name(w346) -> ("Motor 1 P Gains"=w350:T6, "Motor 1 V Gains"=w351:T6, "Velocity Limits"=w352:cluster{"output high":dbl, "output low":dbl}, "Duty Cycle Limits"=w353:cluster{"output high":dbl, "output low":dbl})
              n158 = Absolute Value(x=w334) -> (abs(x)=w336:dbl)
              n159 = Greater?(x=w336, y=w335) -> (0:w339:bool)
              n160 = call-poly <vilib>:"PID.vi"("output range"=w352, "PID gains"=w350, "process variable"=w333, "setpoint"=w329) -> ("output"=w331:dbl)  [unwired: 6 in, 1 out]
              n161 = Add(x=w331, y=w332) -> (x+y=w330:dbl)
              n162 = Greater Or Equal?(x=w331, y=0.0) -> (x >= y?=w356:bool)
              n163 = Select(t=enum8{"Clockwise", "Counterclockwise"}."Clockwise" ("Mod1/Drive Direction"), s=w356, f=enum8{"Clockwise", "Counterclockwise"}."Counterclockwise" ("Mod1/Drive Direction")) -> (s? t:f=w344:enum8{"Clockwise", "Counterclockwise"})
              n164 = call-poly <vilib>:"PID.vi"("output range"=w353, "PID gains"=w351, "process variable"=w341, "setpoint"=w330) -> ("output"=w348:dbl)  [unwired: 6 in, 1 out]
              n165 = Absolute Value(x=w348) -> (abs(x)=w349:dbl)
              n166 = To Fixed-Point(fixed-point type=fxp<+,32,0> 0.0 ("Duty Cycle 1"), number=w349) -> (fixed-point=w355:fxp<+,32,0>)
              n167 = Select(t=w355, s=w343, f=fxp<+,32,0> 0.0 ("Duty Cycle 1")) -> (s? t:f=w338:fxp<+,32,0>)
              n168 = Select(t=w338, s=w339, f=fxp<+,32,0> 0.0 ("Duty Cycle 1")) -> (s? t:f=w337:fxp<+,32,0>)
            }
            frame 1 {
              n169 = Unbundle By Name(w375) -> ("Motor 2 Variables"=w376:T7)
              n170 = Subtract(x=w359, y=w363) -> (x-y=w368:dbl)
              n171 = Unbundle By Name(w376) -> ("Motor 2 P Gains"=w380:T6, "Motor 2 V Gains"=w381:T6, "Velocity Limits"=w383:cluster{"output high":dbl, "output low":dbl}, "Duty Cycle Limits"=w382:cluster{"output high":dbl, "output low":dbl})
              n172 = Absolute Value(x=w368) -> (abs(x)=w367:dbl)
              n173 = Greater?(x=w367, y=w366) -> (0:w369:bool)
              n174 = call-poly <vilib>:"PID.vi"("output range"=w383, "PID gains"=w380, "process variable"=w363, "setpoint"=w359) -> ("output"=w361:dbl)  [unwired: 6 in, 1 out]
              n175 = Add(x=w361, y=w362) -> (x+y=w360:dbl)
              n176 = Greater Or Equal?(x=w361, y=0.0) -> (x >= y?=w386:bool)
              n177 = Select(t=enum8{"Clockwise", "Counterclockwise"}."Counterclockwise" ("Mod1/Drive Direction"), s=w386, f=enum8{"Clockwise", "Counterclockwise"}."Clockwise" ("Mod1/Drive Direction")) -> (s? t:f=w374:enum8{"Clockwise", "Counterclockwise"})
              n178 = call-poly <vilib>:"PID.vi"("output range"=w382, "PID gains"=w381, "process variable"=w371, "setpoint"=w360) -> ("output"=w378:dbl)  [unwired: 6 in, 1 out]
              n179 = Absolute Value(x=w378) -> (abs(x)=w379:dbl)
              n180 = To Fixed-Point(fixed-point type=fxp<+,32,0> 0.0 ("Duty Cycle 1"), number=w379) -> (fixed-point=w385:fxp<+,32,0>)
              n181 = Select(t=w385, s=w373, f=fxp<+,32,0> 0.0 ("Duty Cycle 1")) -> (s? t:f=w365:fxp<+,32,0>)
              n182 = Select(t=w365, s=w369, f=fxp<+,32,0> 0.0 ("Duty Cycle 1")) -> (s? t:f=w364:fxp<+,32,0>)
            }
            frame 2 {
              n183 = Unbundle By Name(w405) -> ("Motor 3 Variables"=w406:T8)
              n184 = Subtract(x=w389, y=w393) -> (x-y=w398:dbl)
              n185 = Unbundle By Name(w406) -> ("Motor 3 P Gains"=w413:T6, "Motor 3 V Gains"=w412:T6, "Velocity Limits"=w415:cluster{"output high":dbl, "output low":dbl}, "Duty Cycle Limits"=w414:cluster{"output high":dbl, "output low":dbl})
              n186 = Absolute Value(x=w398) -> (abs(x)=w397:dbl)
              n187 = Greater?(x=w397, y=w396) -> (0:w399:bool)
              n188 = call-poly <vilib>:"PID.vi"("output range"=w415, "PID gains"=w413, "process variable"=w393, "setpoint"=w389) -> ("output"=w391:dbl)  [unwired: 6 in, 1 out]
              n189 = Add(x=w391, y=w392) -> (x+y=w390:dbl)
              n190 = Greater Or Equal?(x=w391, y=0.0) -> (x >= y?=w416:bool)
              n191 = Select(t=enum8{"Clockwise", "Counterclockwise"}."Counterclockwise" ("Mod1/Drive Direction"), s=w416, f=enum8{"Clockwise", "Counterclockwise"}."Clockwise" ("Mod1/Drive Direction")) -> (s? t:f=w404:enum8{"Clockwise", "Counterclockwise"})
              n192 = call-poly <vilib>:"PID.vi"("output range"=w414, "PID gains"=w412, "process variable"=w401, "setpoint"=w390) -> ("output"=w410:dbl)  [unwired: 6 in, 1 out]
              n193 = Absolute Value(x=w410) -> (abs(x)=w411:dbl)
              n194 = To Fixed-Point(fixed-point type=fxp<+,32,0> 0.0 ("Duty Cycle 1"), number=w411) -> (fixed-point=w407:fxp<+,32,0>)
              n195 = Select(t=w407, s=w403, f=fxp<+,32,0> 0.0 ("Duty Cycle 1")) -> (s? t:f=w395:fxp<+,32,0>)
              n196 = Select(t=w395, s=w399, f=fxp<+,32,0> 0.0 ("Duty Cycle 1")) -> (s? t:f=w394:fxp<+,32,0>)
            }
            frame 3 {
              n197 = Unbundle By Name(w435) -> ("Motor 4 Variables"=w436:T9)
              n198 = Subtract(x=w422, y=w423) -> (x-y=w428:dbl)
              n199 = Unbundle By Name(w436) -> ("Motor 4 P Gains"=w442:T6, "Motor 4 V Gains"=w443:T6, "Velocity Limits"=w440:cluster{"output high":dbl, "output low":dbl}, "Duty Cycle Limits"=w441:cluster{"output high":dbl, "output low":dbl})
              n200 = Absolute Value(x=w428) -> (abs(x)=w427:dbl)
              n201 = Greater?(x=w427, y=w426) -> (0:w429:bool)
              n202 = call-poly <vilib>:"PID.vi"("output range"=w440, "PID gains"=w442, "process variable"=w423, "setpoint"=w422) -> ("output"=w420:dbl)  [unwired: 6 in, 1 out]
              n203 = Add(x=w420, y=w421) -> (x+y=w419:dbl)
              n204 = Greater Or Equal?(x=w420, y=0.0) -> (x >= y?=w446:bool)
              n205 = Select(t=enum8{"Clockwise", "Counterclockwise"}."Counterclockwise" ("Mod1/Drive Direction"), s=w446, f=enum8{"Clockwise", "Counterclockwise"}."Clockwise" ("Mod1/Drive Direction")) -> (s? t:f=w434:enum8{"Clockwise", "Counterclockwise"})
              n206 = call-poly <vilib>:"PID.vi"("output range"=w441, "PID gains"=w443, "process variable"=w431, "setpoint"=w419) -> ("output"=w438:dbl)  [unwired: 6 in, 1 out]
              n207 = Absolute Value(x=w438) -> (abs(x)=w439:dbl)
              n208 = To Fixed-Point(fixed-point type=fxp<+,32,0> 0.0 ("Duty Cycle 1"), number=w439) -> (fixed-point=w445:fxp<+,32,0>)
              n209 = Select(t=w445, s=w433, f=fxp<+,32,0> 0.0 ("Duty Cycle 1")) -> (s? t:f=w425:fxp<+,32,0>)
              n210 = Select(t=w425, s=w429, f=fxp<+,32,0> 0.0 ("Duty Cycle 1")) -> (s? t:f=w424:fxp<+,32,0>)
            }
            frame 4 {
              n211 = Unbundle By Name(w465) -> ("Motor 5 Variables"=w466:T10)
              n212 = Subtract(x=w452, y=w453) -> (x-y=w456:dbl)
              n213 = Unbundle By Name(w466) -> ("Motor 5 P Gains"=w470:T6, "Motor 5 V Gains"=w473:T6, "Velocity Limits"=w471:cluster{"output high":dbl, "output low":dbl}, "Duty Cycle Limits"=w472:cluster{"output high":dbl, "output low":dbl})
              n214 = Absolute Value(x=w456) -> (abs(x)=w457:dbl)
              n215 = Greater?(x=w457, y=w458) -> (0:w459:bool)
              n216 = call-poly <vilib>:"PID.vi"("output range"=w471, "PID gains"=w470, "process variable"=w453, "setpoint"=w452) -> ("output"=w450:dbl)  [unwired: 6 in, 1 out]
              n217 = Add(x=w450, y=w451) -> (x+y=w449:dbl)
              n218 = Greater Or Equal?(x=w450, y=0.0) -> (x >= y?=w476:bool)
              n219 = Select(t=enum8{"Clockwise", "Counterclockwise"}."Counterclockwise" ("Mod1/Drive Direction"), s=w476, f=enum8{"Clockwise", "Counterclockwise"}."Clockwise" ("Mod1/Drive Direction")) -> (s? t:f=w464:enum8{"Clockwise", "Counterclockwise"})
              n220 = call-poly <vilib>:"PID.vi"("output range"=w472, "PID gains"=w473, "process variable"=w461, "setpoint"=w449) -> ("output"=w468:dbl)  [unwired: 6 in, 1 out]
              n221 = Absolute Value(x=w468) -> (abs(x)=w469:dbl)
              n222 = To Fixed-Point(fixed-point type=fxp<+,32,0> 0.0 ("Duty Cycle 1"), number=w469) -> (fixed-point=w475:fxp<+,32,0>)
              n223 = Select(t=w475, s=w463, f=fxp<+,32,0> 0.0 ("Duty Cycle 1")) -> (s? t:f=w455:fxp<+,32,0>)
              n224 = Select(t=w455, s=w459, f=fxp<+,32,0> 0.0 ("Duty Cycle 1")) -> (s? t:f=w454:fxp<+,32,0>)
            }
          }
        }
      }
    }
    n225 = Divide(x=w83, y=1000.0) -> (x/y=w41:dbl)
    n226 = Build Array (concatenate)(w41, w39) -> (w40:dbl[])
    n227 = Initialize Array(0.0 ("element"), 1024 ("dimension size"), 11 ("dimension size")) -> (w47:dbl[][])
    n228 = feedback #8(w47) -> (w48:dbl[][])
    n229 = feedback #9(0 ("y")) -> (w66:i32)
    n230 = Quotient & Remainder(x=w66, y=1024) -> (x-y*floor(x/y)=w54:i32)  [unwired: 1 out]
    n231 = for {
      tunnel: w40 -> [w551] mode=indexing
      tunnel: w54 -> [w550]
      shift-right: [w552] -> w53
      shift-left: w48 -> [w553]
      i -> [w549]
      n232 = Replace Array Subset(array=w553, new element=w551, index (row)=w550, index (col)=w549) -> (w552:dbl[][])
    }
    n233 = Equal?(x=w54, y=1023) -> (x = y?=w71:bool)
    n234 = case shown="True" w71 {
      tunnel: w54 -> [w555 w559]
      tunnel: [w555 w559] -> w67
      tunnel: w53 -> [w554 w557]
      tunnel: [w554 w558] -> w49
      tunnel: w47 -> [_ w558]
      tunnel: w46 -> [_ w556]
      frame False {
      }
      frame True {
        n235 = Enqueue Element(queue=w556, element=w557) -> ()  [unwired: 2 in, 3 out]
      }
    }
    n236 = feedback-in #8(w49) -> ()
    n237 = Increment(x=w67) -> (x+1=w68:i32)
    n238 = feedback-in #9(w68) -> ()
    n239 = shared-variable "My Computer\\Shared_Variables.lvlib\\Stop"() -> (w23:bool)  [unwired: 1 in, 1 out]
    n240 = Or(x="stop", y=w23) -> (x .or. y?=w25:bool)
    n241 = Index Array(array=w32) -> (element #1=w31:fxp<+,32,0>, element #2=w30:fxp<+,32,0>, element #3=w29:fxp<+,32,0>, element #4=w28:fxp<+,32,0>, element #5=w27:fxp<+,32,0>)  [unwired: 5 in]
    n242 = Index Array(array=w38) -> (element #1=w37:enum8{"Clockwise", "Counterclockwise"}, element #2=w35:enum8{"Clockwise", "Counterclockwise"}, element #3=w36:enum8{"Clockwise", "Counterclockwise"}, element #4=w34:enum8{"Clockwise", "Counterclockwise"}, element #5=w33:enum8{"Clockwise", "Counterclockwise"})  [unwired: 5 in]
    n243 = xnode "Read/Write Control"("FPGA VI Reference In"=w82, "Duty Cycle 1"=w31, "Duty Cycle 2"=w30, "Duty Cycle 3"=w29, "Duty Cycle 4"=w28, "Duty Cycle 5"=w27, "Mod1/Drive Direction"=w37, "Mod1/Drive Direction 2"=w35, "Mod1/Drive Direction 3"=w36, "Mod1/Drive Direction 4"=w34, "Mod1/Drive Direction 5"=w33, "Stop"=w25, "Velocity Interval (uSec)"=fxp<+/-,40,24> 5000.0) -> ("FPGA VI Reference Out"=w89:refnum<k20>)  [unwired: 1 in, 1 out]
    n244 = node-c288() -> ()  [unwired: 1 in, 1 out]
  }
  n245 = while {
    tunnel: w9 -> [w564]
    tunnel: [w563] -> w8
    shift-right: [w561] -> _
    shift-left: dbl[][] [] -> [w562]
    stop <- w560 stop-if-true
    n246 = Get Queue Status(queue=w564) -> (queue out=w563:refnum<queue>, # elements in queue=w567:i32)  [unwired: 2 in, 6 out]
    n247 = Greater?(x=w567, y=0) -> (0:w565:bool)
    n248 = case shown="False" w565 {
      tunnel: w564 -> [_ w570]
      tunnel: [w568 w569] -> w561
      tunnel: w562 -> [w568 _]
      frame False {
      }
      frame True {
        n249 = Dequeue Element(queue=w570) -> (element=w569:dbl[][])  [unwired: 2 in, 3 out]
      }
    }
    "appended array" <- w561
    n250 = shared-variable "My Computer\\Shared_Variables.lvlib\\Stop"() -> (w560:bool)  [unwired: 1 in, 1 out]
  }
  n251 = Release Queue(queue=w8) -> ()  [unwired: 2 in, 3 out]
  n252 = node-c288(w3) -> ()  [unwired: 1 out]
  n253 = xnode "Close FPGA VI Reference"("FPGA VI Reference In"=w12) -> ()  [unwired: 1 in, 1 out]
